vi "Override Error.vi"(10 "Error":errorcluster, 11 "Base Event Actor in":refnum<class "Base Event Actor.lvclass">) -> (3 "Base Event Actor out":refnum<class "Base Event Actor.lvclass">)   [LabVIEW 2021, in "jettl.lvlib" / "Base Event Actor.lvclass"]
uses:
  Base Event Actor.lvclass
  Base Event Actor.lvclass/Base Event Actor.ctl
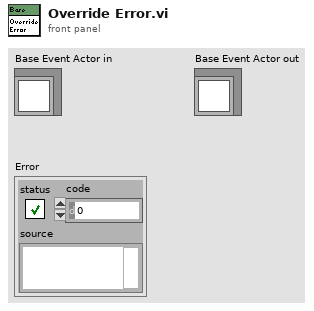
[diagram p1: front panel]
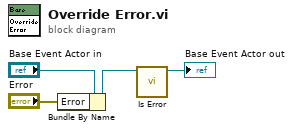
[diagram p0: block diagram]
diagram:
  n1 = Bundle By Name(cluster="Base Event Actor in", "Error"="Error") -> (w2:refnum<class "Base Event Actor.lvclass">)
  n2 = call "Is Error.vi"("Base Event Actor in"=w2) -> ("Base Event Actor out"=→"Base Event Actor out":refnum<class "Base Event Actor.lvclass">)  [unwired: 10 in]
